vi "Clavier virtuel.vi"(7 "Mode":enum16{"Normal", "Password"}(ring), 8 "error in (no error)":errorcluster, 11 "Str Refnum":refnum<vi>) -> (0 "error out":errorcluster)   [LabVIEW 2012]
doc: "Virutal keyboard ( click on \"-->\" to exit)"
uses:
  <vilib>/Utility/miscctls.llb/LVPointTypeDef.ctl
  <vilib>/Utility/miscctls.llb/LVPositionTypeDef.ctl
panel:
  out "String":string
  out "SHIFT2":bool
  out "SHIFT1":bool
  out "CAPS LOCK":bool
  in  "E3":bool
  in  "E4":bool
  in  "E11":bool
  in  "E6":bool
  in  "E1":bool
  in  "E9":bool
  in  "E5":bool
  in  "E8":bool
  in  "E7":bool
  in  "E12":bool
  in  "E2":bool
  in  "E10":bool
  in  "D3":bool
  in  "D7":bool
  in  "D11":bool
  in  "D1":bool
  in  "D5":bool
  in  "D9":bool
  in  "D4":bool
  in  "D8":bool
  in  "D12":bool
  in  "D2":bool
  in  "D6":bool
  in  "D10":bool
  in  "C2":bool
  in  "C12":bool
  in  "C4":bool
  in  "C10":bool
  in  "C6":bool
  in  "C8":bool
  in  "C1":bool
  in  "C11":bool
  in  "C3":bool
  in  "C9":bool
  in  "C5":bool
  in  "C7":bool
  in  "B1":bool
  in  "B6":bool
  in  "B12":bool
  in  "B11":bool
  in  "B9":bool
  in  "B2":bool
  in  "B5":bool
  in  "B3":bool
  in  "B4":bool
  in  "B7":bool
  in  "B8":bool
  in  "B10":bool
  in  "A12":bool
  in  "A11":bool
  in  "A7":bool
  in  "A9":bool
  in  "A10":bool
  in  "A8":bool
  in  "A6":bool
  in  "A3":bool
  in  "A4":bool
  in  "A5":bool
  in  "A2":bool
  in  "A1":bool
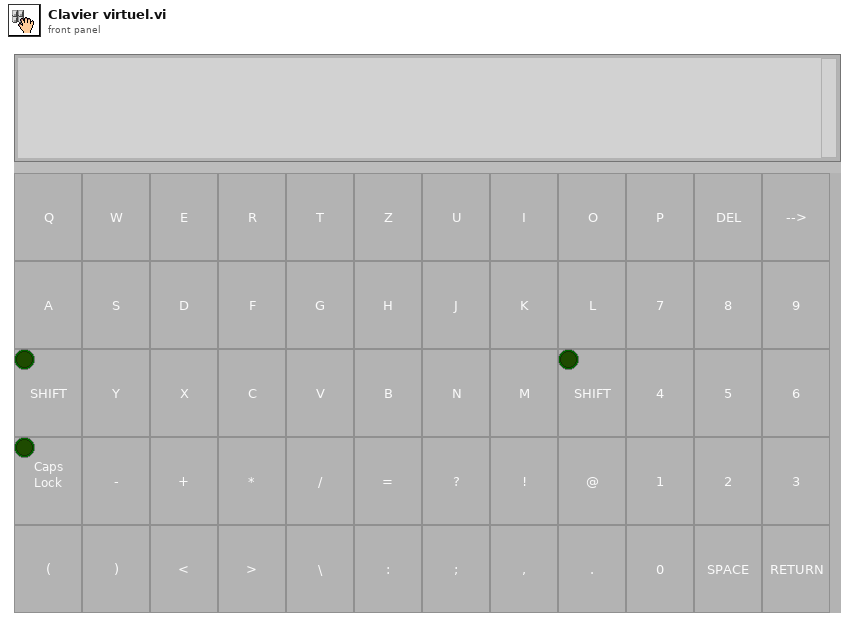
[diagram p1: front panel]
types:
  T1 = typedef "LVPositionTypeDef.ctl" = cluster{"Left":i32, "Top":i32}
  T2 = typedef "LVPointTypeDef.ctl" = cluster{"Horizontal":i16, "Vertical":i16}
  T3 = typedef "LVBoundsTypeDef.ctl" = cluster{"Width":u32, "Height":u32}
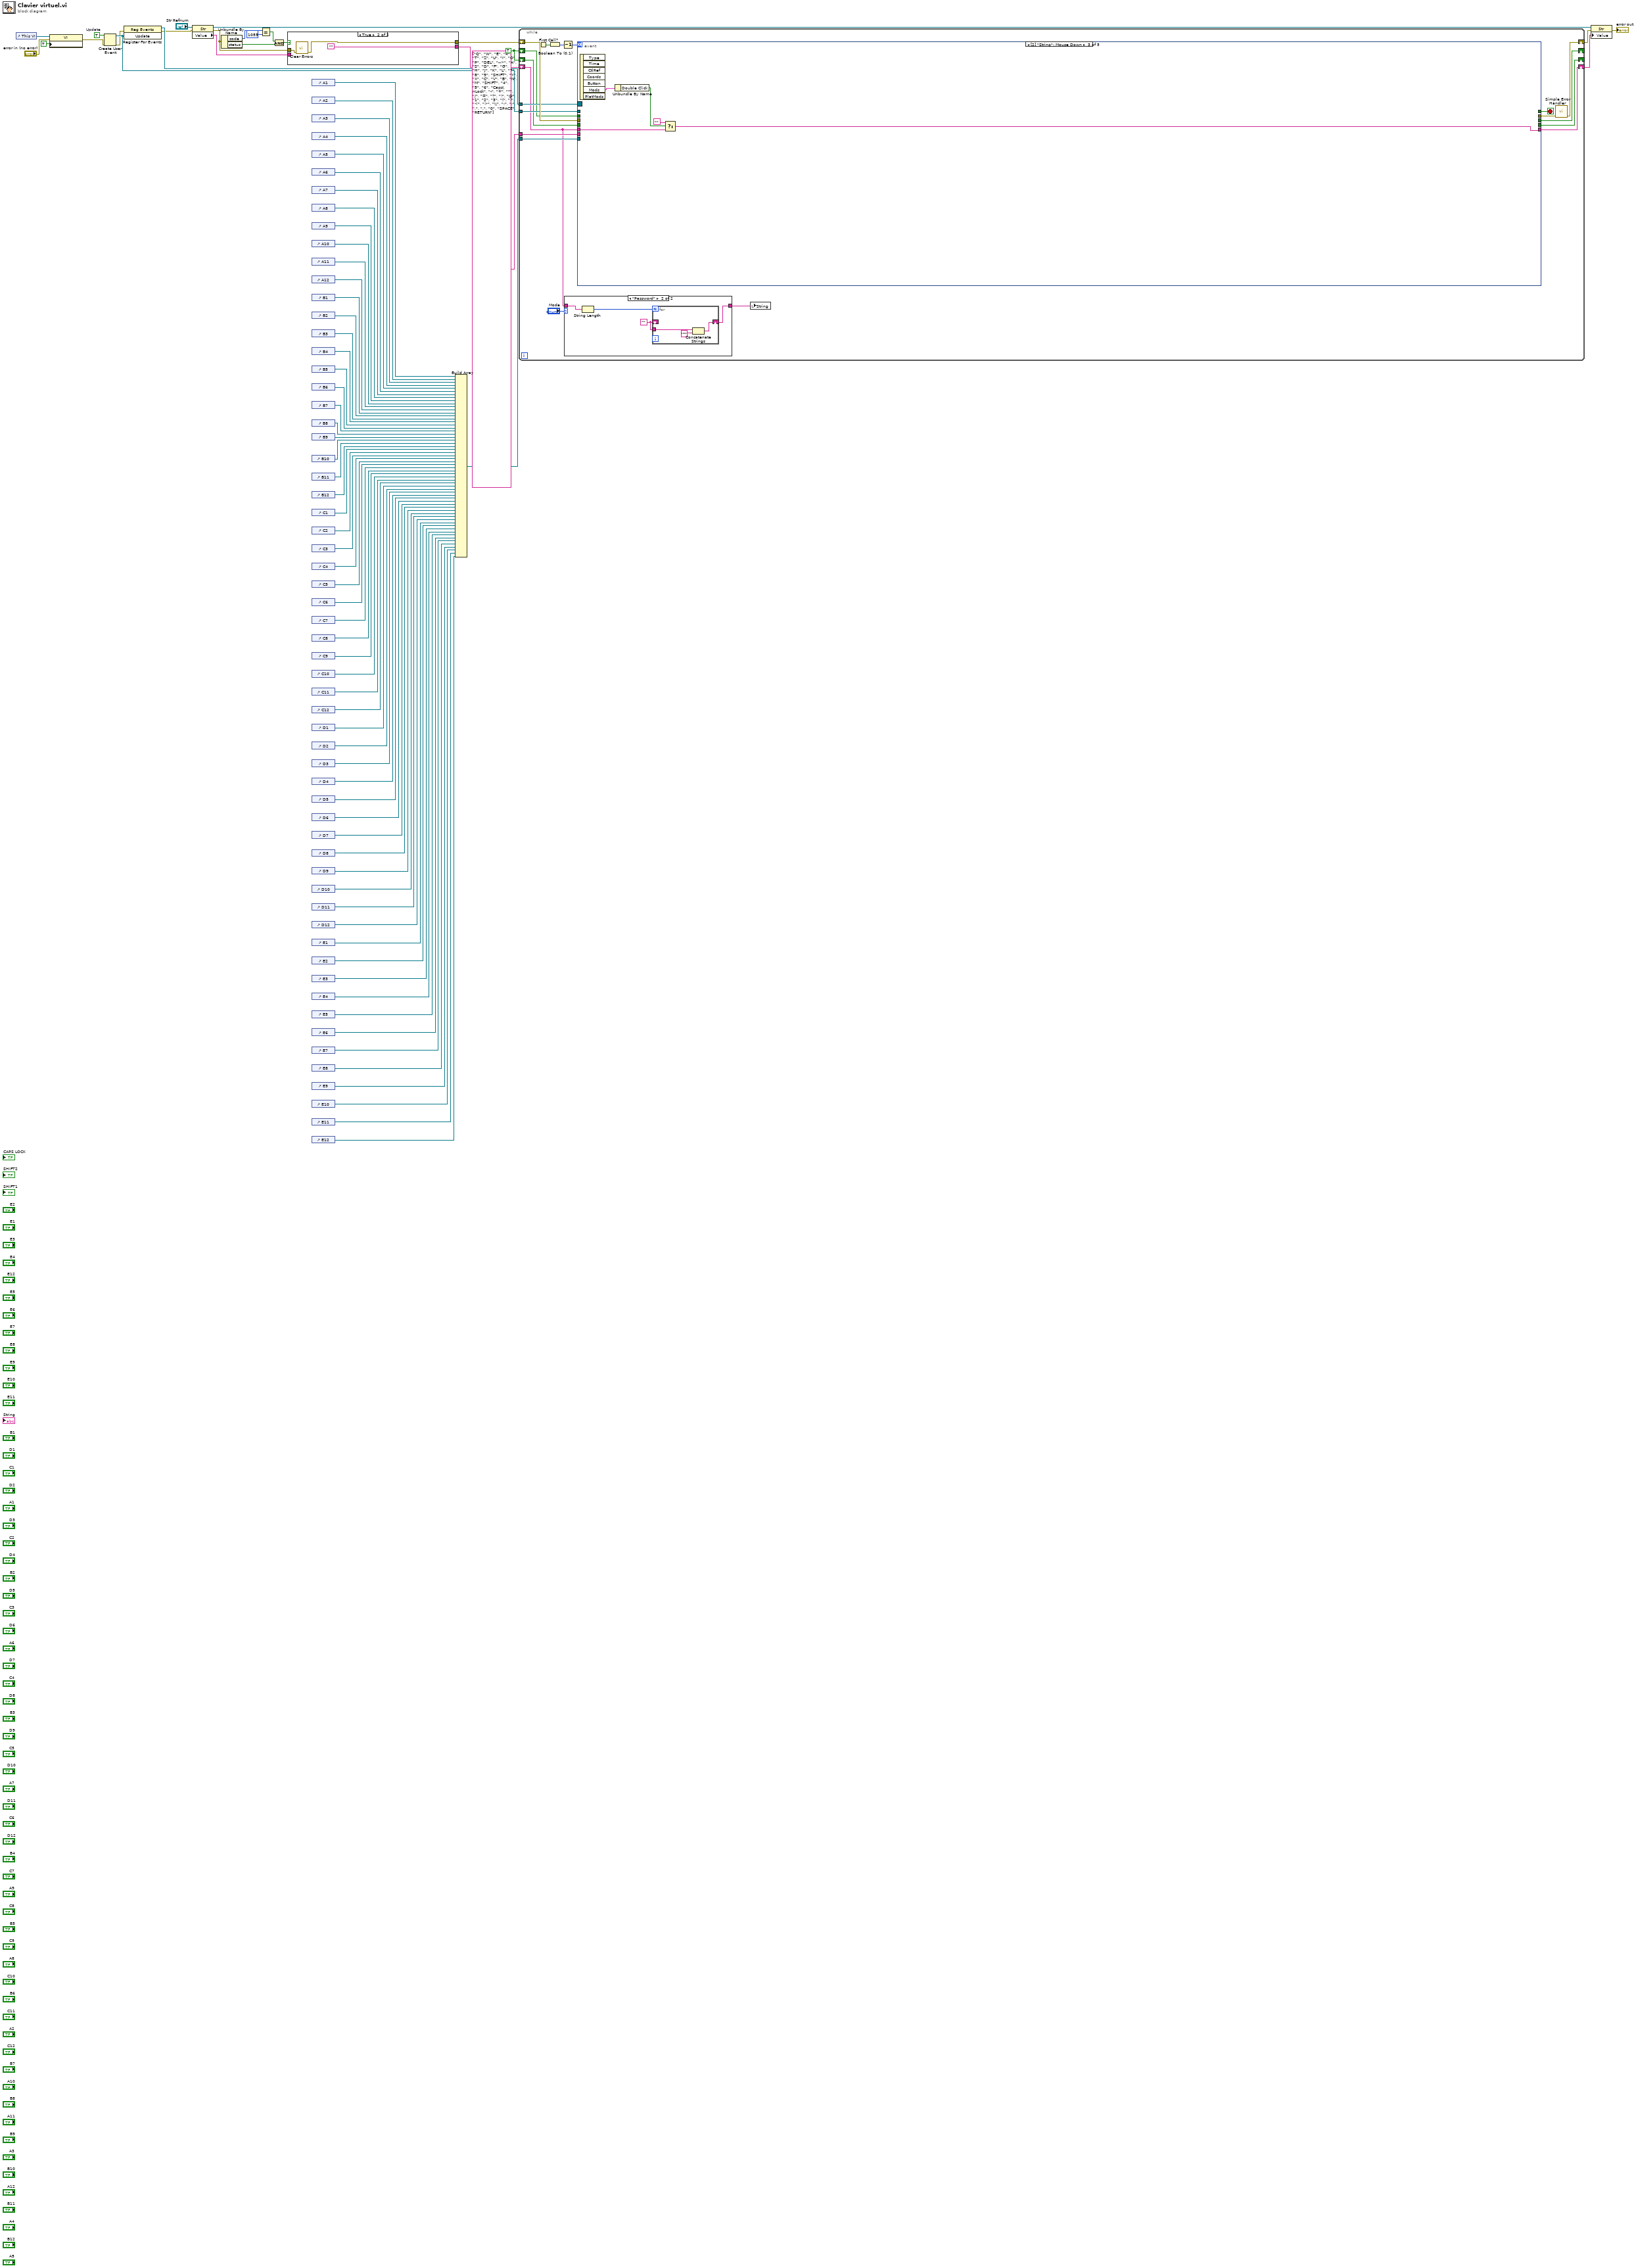
[diagram p0: block diagram]
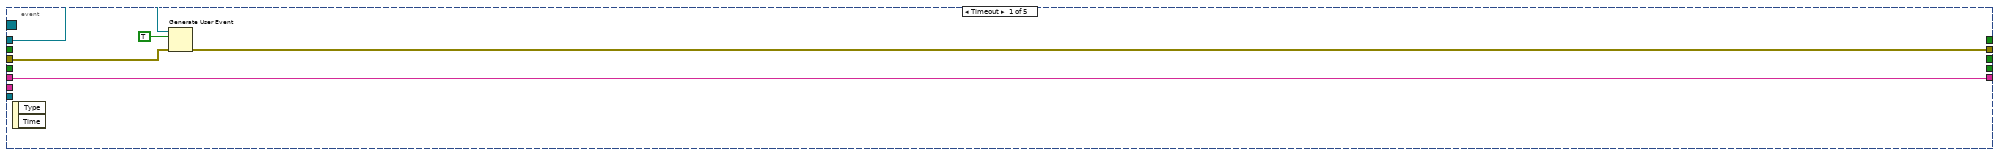
[diagram p4: hidden frame]
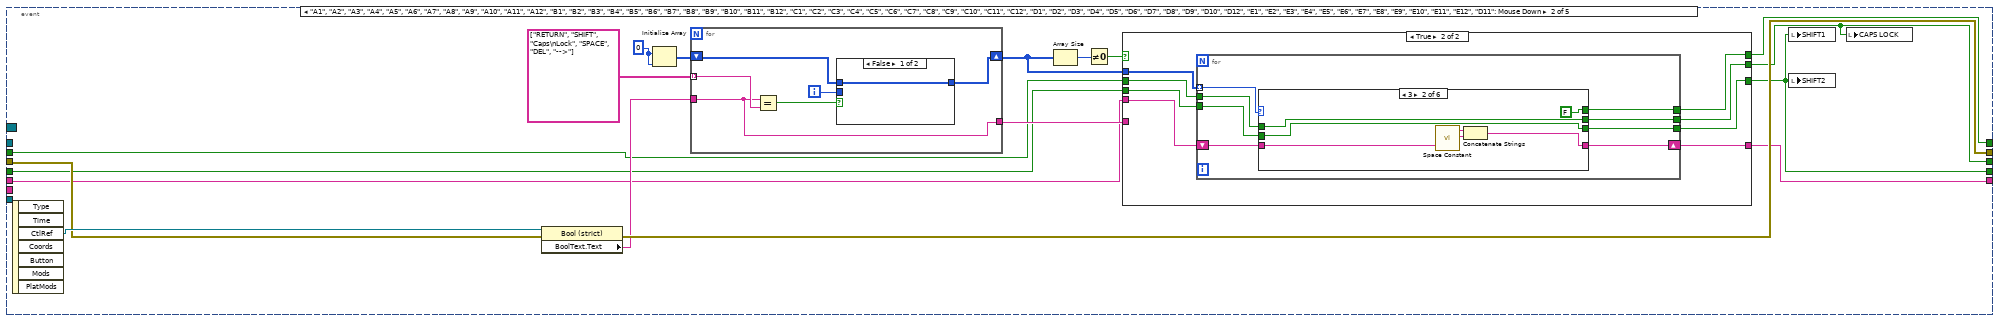
[diagram p5: hidden frame]
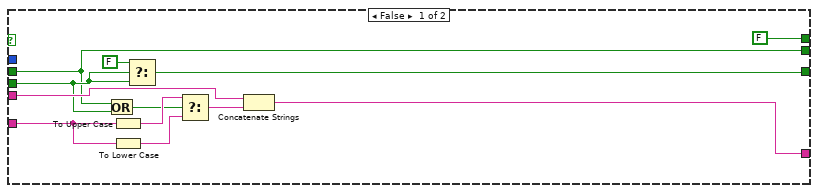
[diagram p6: hidden frame]
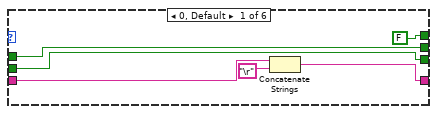
[diagram p7: hidden frame]
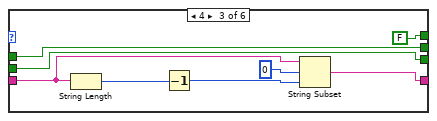
[diagram p8: hidden frame]
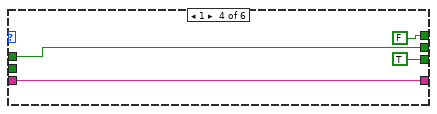
[diagram p9: hidden frame]
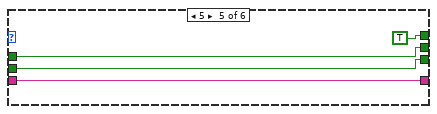
[diagram p10: hidden frame]
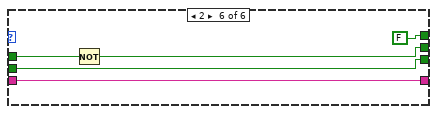
[diagram p11: hidden frame]
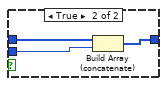
[diagram p12: hidden frame]
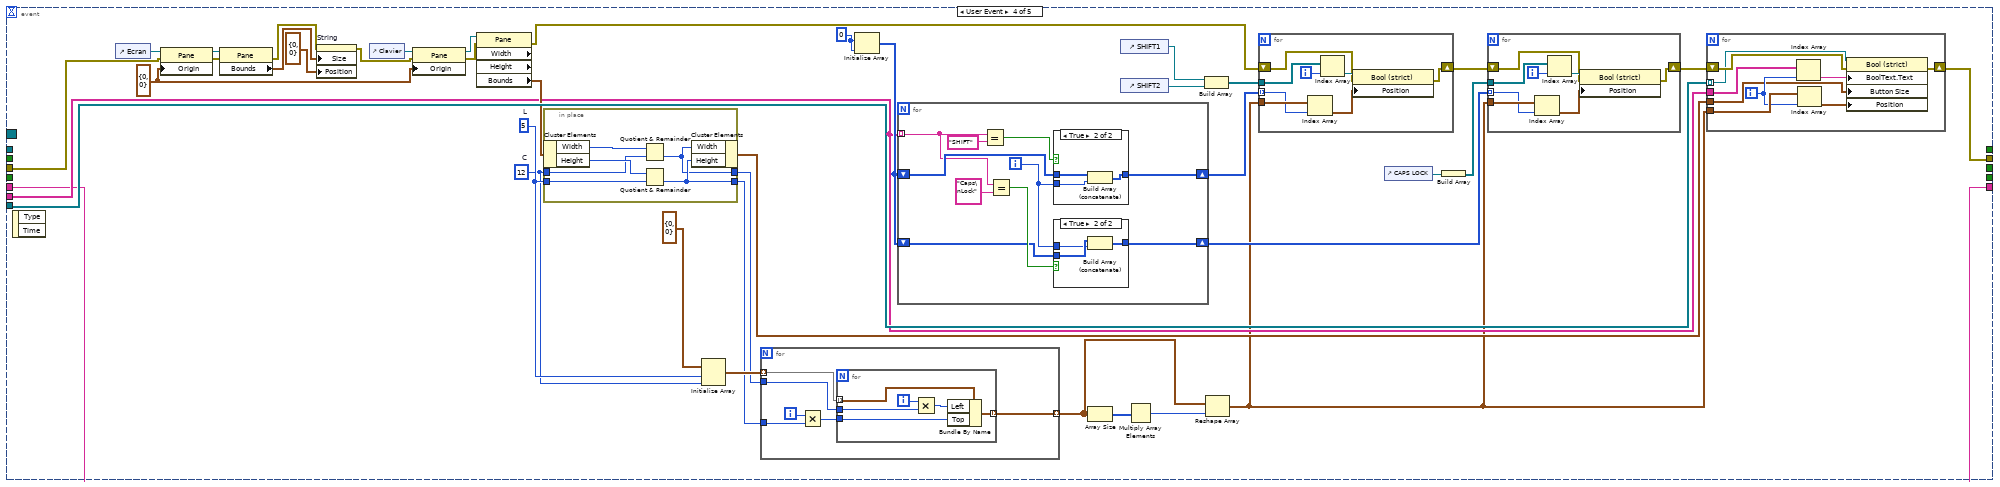
[diagram p13: hidden frame]
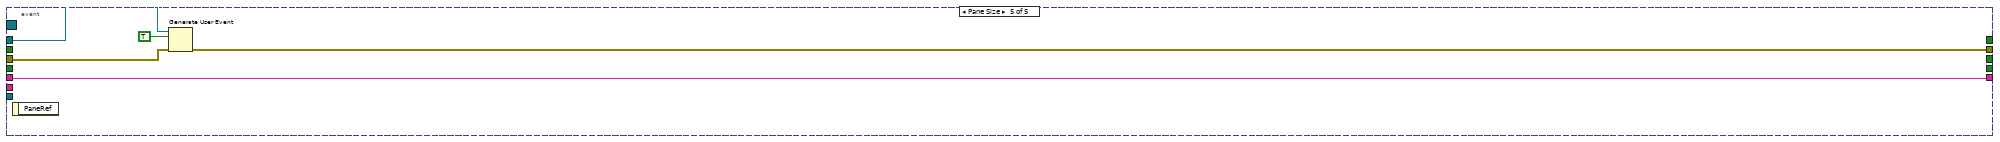
[diagram p16: hidden frame]
diagram:
  w21 = TRUE
  w73 = TRUE  # Update
  n1 = control-ref of="This VI"() -> (w4:refnum<vi>)
  n2 = property class="VI"(reference=w4, error in="error in (no error)", "Front Panel.IsFrontmost"=TRUE ("Front Panel Window:Is Frontmost")) -> (error out=w2:errorcluster)  [unwired: 1 out]
  n3 = Create User Event(user event datatype=w73, error in=w2) -> (user event=w72:refnum<user-event>, error out=w11:errorcluster)
  n4 = register-events(error in=w11, w72) -> (reference out=w71:refnum<event-registration>, error out=w10:errorcluster)  [unwired: 1 in]
  n5 = property class="Str"(reference="Str Refnum", error in=w10) -> (reference out=w16:refnum<vi>, error out=w13:errorcluster, "Value"=w15:string)
  n6 = Unbundle By Name(w13) -> ("code"=w8:i32, "status"=w7:bool)
  n7 = Equal?(x=w8, y=1055) -> (x = y?=w6:bool)
  n8 = And(x=w6, y=w7) -> (x .and. y?=w5:bool)
  n9 = case shown="True" w5 {
    tunnel: w13 -> [w87 w91]
    tunnel: w15 -> [w88 _]
    tunnel: [w88 ""] -> w14
    tunnel: [w87 w90] -> w12
    frame False {
    }
    frame True {
      n10 = call <vilib>:"Clear Errors.vi"("error in (no error)"=w91) -> ("error out"=w90:errorcluster)  [unwired: 6 in]
    }
  }
  n11 = control-ref of="A1"() -> (w82:refnum<vi>)
  n12 = control-ref of="A2"() -> (w83:refnum<vi>)
  n13 = control-ref of="A3"() -> (w84:refnum<vi>)
  n14 = control-ref of="A4"() -> (w85:refnum<vi>)
  n15 = control-ref of="A5"() -> (w86:refnum<vi>)
  n16 = control-ref of="A6"() -> (w81:refnum<vi>)
  n17 = control-ref of="A7"() -> (w80:refnum<vi>)
  n18 = control-ref of="A8"() -> (w79:refnum<vi>)
  n19 = control-ref of="A9"() -> (w78:refnum<vi>)
  n20 = control-ref of="A10"() -> (w77:refnum<vi>)
  n21 = control-ref of="A11"() -> (w76:refnum<vi>)
  n22 = control-ref of="A12"() -> (w75:refnum<vi>)
  n23 = control-ref of="B1"() -> (w69:refnum<vi>)
  n24 = control-ref of="B2"() -> (w68:refnum<vi>)
  n25 = control-ref of="B3"() -> (w67:refnum<vi>)
  n26 = control-ref of="B4"() -> (w66:refnum<vi>)
  n27 = control-ref of="B5"() -> (w65:refnum<vi>)
  n28 = control-ref of="B6"() -> (w64:refnum<vi>)
  n29 = control-ref of="B7"() -> (w63:refnum<vi>)
  n30 = control-ref of="B8"() -> (w62:refnum<vi>)
  n31 = control-ref of="B9"() -> (w61:refnum<vi>)
  n32 = control-ref of="B10"() -> (w60:refnum<vi>)
  n33 = control-ref of="B11"() -> (w59:refnum<vi>)
  n34 = control-ref of="B12"() -> (w58:refnum<vi>)
  n35 = control-ref of="C1"() -> (w57:refnum<vi>)
  n36 = control-ref of="C2"() -> (w56:refnum<vi>)
  n37 = control-ref of="C3"() -> (w55:refnum<vi>)
  n38 = control-ref of="C4"() -> (w54:refnum<vi>)
  n39 = control-ref of="C5"() -> (w53:refnum<vi>)
  n40 = control-ref of="C6"() -> (w52:refnum<vi>)
  n41 = control-ref of="C7"() -> (w51:refnum<vi>)
  n42 = control-ref of="C8"() -> (w50:refnum<vi>)
  n43 = control-ref of="C9"() -> (w49:refnum<vi>)
  n44 = control-ref of="C10"() -> (w48:refnum<vi>)
  n45 = control-ref of="C11"() -> (w47:refnum<vi>)
  n46 = control-ref of="C12"() -> (w46:refnum<vi>)
  n47 = control-ref of="D1"() -> (w45:refnum<vi>)
  n48 = control-ref of="D2"() -> (w44:refnum<vi>)
  n49 = control-ref of="D3"() -> (w43:refnum<vi>)
  n50 = control-ref of="D4"() -> (w42:refnum<vi>)
  n51 = control-ref of="D5"() -> (w41:refnum<vi>)
  n52 = control-ref of="D6"() -> (w40:refnum<vi>)
  n53 = control-ref of="D7"() -> (w39:refnum<vi>)
  n54 = control-ref of="D8"() -> (w38:refnum<vi>)
  n55 = control-ref of="D9"() -> (w37:refnum<vi>)
  n56 = control-ref of="D10"() -> (w36:refnum<vi>)
  n57 = control-ref of="D11"() -> (w35:refnum<vi>)
  n58 = control-ref of="D12"() -> (w34:refnum<vi>)
  n59 = control-ref of="E1"() -> (w33:refnum<vi>)
  n60 = control-ref of="E2"() -> (w32:refnum<vi>)
  n61 = control-ref of="E3"() -> (w31:refnum<vi>)
  n62 = control-ref of="E4"() -> (w30:refnum<vi>)
  n63 = control-ref of="E5"() -> (w29:refnum<vi>)
  n64 = control-ref of="E6"() -> (w28:refnum<vi>)
  n65 = control-ref of="E7"() -> (w27:refnum<vi>)
  n66 = control-ref of="E8"() -> (w26:refnum<vi>)
  n67 = control-ref of="E9"() -> (w25:refnum<vi>)
  n68 = control-ref of="E10"() -> (w24:refnum<vi>)
  n69 = control-ref of="E11"() -> (w23:refnum<vi>)
  n70 = control-ref of="E12"() -> (w22:refnum<vi>)
  n71 = Build Array(w82, w83, w84, w85, w86, w81, w80, w79, w78, w77, w76, w75, w69, w68, w67, w66, w65, w64, w63, w62, w61, w60, w59, w58, w57, w56, w55, w54, w53, w52, w51, w50, w49, w48, w47, w46, w45, w44, w43, w42, w41, w40, w39, w38, w37, w36, w35, w34, w33, w32, w31, w30, w29, w28, w27, w26, w25, w24, w23, w22) -> (w70:refnum<vi>[])
  n72 = while {
    shift-right: [w110] -> w18
    shift-left: w14 -> [w92]
    shift-right: [w95] -> w20
    shift-left: w12 -> [w108]
    tunnel: w70 -> [w104]
    tunnel: string[] ["Q", "W", "E", "R", "T", "Z", "U", "I", "O", "P", "DEL", "-->", "A", "S", "D", "F", "G", "H", "J", "K", "L", "7", "8", "9", "SHIFT", "Y", "X", "C", "V", "B", "N", "M", "SHIFT", "4", "5", "6", "Caps\nLock", "-", "+", "*", "/", "=", "?", "!", "@", "1", "2", "3", "(", ")", "<", ">", "\\", ":", ";", ",", ".", "0", "SPACE", "RETURN"] -> [w103]
    tunnel: w72 -> [w102]
    tunnel: w71 -> [w101]
    shift-right: [w97] -> _
    shift-left: w21 -> [w99]
    shift-right: [w96] -> _
    shift-left: w21 -> [w98]
    stop <- w109 stop-if-true
    n73 = First Call?() -> (First Call?: T/F=w106:bool)
    n74 = Boolean To (0,1)(Boolean=w106) -> (0, 1=w107:i16)
    n75 = Decrement(x=w107) -> (x-1=w105:i16)
    n76 = case shown="\"Password\"" "Mode" {
      tunnel: w92 -> [w111 w115]
      tunnel: [w111 w114] -> w93
      frame "Normal", Default {
      }
      frame "Password" {
        w113 = ""
        n77 = String Length(string=w115) -> (length=w112:i32)
        n78 = for {
          N: w112 -> [_]
          shift-right: [w117] -> w114
          shift-left: w113 -> [_]
          tunnel: w113 -> [w118]
          n79 = Concatenate Strings(w118, "*") -> (w117:string)
        }
      }
    }
    n80 = event shown="[2] \"String\": Mouse Down" {
      selector: w101 -> [_ _ _ _ _]
      dyn-events: _ -> [_ _ _ _ _]
      timeout: w105 -> [_ _ _ _ _]
      tunnel: w92 -> [w119 w128 w215 w218 w319]
      tunnel: [w119 w130 w213 w218 w319] -> w110
      tunnel: [_ w129 _ _ _] -> w109
      tunnel: w108 -> [w121 w140 _ w252 w321]
      tunnel: [w120 w139 _ w250 w320] -> w100
      tunnel: w104 -> [_ _ _ w251 _]
      tunnel: w103 -> [_ _ _ w230 _]
      tunnel: w102 -> [w122 _ _ _ w322]
      tunnel: w99 -> [_ w127 _ _ _]
      tunnel: w98 -> [_ w125 _ _ _]
      tunnel: [_ w126 _ _ _] -> w97
      tunnel: [_ w124 _ _ _] -> w96
      event Timeout {
        n81 = event-data() -> ()  [unwired: 1 in, 2 out]
        n82 = Generate User Event(user event=w122, event data cluster=TRUE ("event data"), error in=w121) -> (error out=w120:errorcluster)  [unwired: 1 out]
      }
      event "A1", "A2", "A3", "A4", "A5", "A6", "A7", "A8", "A9", "A10", "A11", "A12", "B1", "B2", "B3", "B4", "B5", "B6", "B7", "B8", "B9", "B10", "B11", "B12", "C1", "C2", "C3", "C4", "C5", "C6", "C7", "C8", "C9", "C10", "C11", "C12", "D1", "D2", "D3", "D4", "D5", "D6", "D7", "D8", "D9", "D10", "D12", "E1", "E2", "E3", "E4", "E5", "E6", "E7", "E8", "E9", "E10", "E11", "E12", "D11": Mouse Down {
        w138 = 0
        n83 = event-data() -> ("CtlRef"=w141:refnum<vi>)  [unwired: 1 in, 6 out]
        n84 = property class="Bool (strict)"(reference=w141, error in=w140) -> (error out=w139:errorcluster, "BoolText.Text"=w136:string)  [unwired: 1 out]
        n85 = Initialize Array(w138, w138) -> (w135:i32[])
        n86 = for {
          shift-right: [w206] -> w131
          shift-left: w135 -> [w207]
          tunnel: string[] ["RETURN", "SHIFT", "Caps\nLock", "SPACE", "DEL", "-->"] -> [w208] mode=indexing
          tunnel: w136 -> [w203]
          tunnel: [w203] -> w132
          i -> [w204]
          n87 = Equal?(x=w203, y=w208) -> (x = y?=w205:bool)
          n88 = case shown="False" w205 {
            tunnel: w207 -> [w209 w211]
            tunnel: [w209 w212] -> w206
            tunnel: w204 -> [_ w210]
            frame False {
            }
            frame True {
              n89 = Build Array (concatenate)(w211, w210) -> (w212:i32[])
            }
          }
        }
        n90 = Array Size(array=w131) -> (size(s)=w134:i32)
        n91 = Not Equal To 0?(x=w134) -> (x != 0?=w133:bool)
        n92 = case shown="True" w133 {
          tunnel: w132 -> [w152 _]
          tunnel: w128 -> [w149 w158]
          tunnel: [w148 w160] -> w130
          tunnel: w131 -> [_ w161]
          tunnel: [FALSE w159] -> w129
          tunnel: w127 -> [w142 w157]
          tunnel: [w142 w156] -> w126
          tunnel: w125 -> [w143 w155]
          tunnel: [w145 w154] -> w124
          frame False {
            n93 = Or(x=w142, y=w143) -> (x .or. y?=w144:bool)
            n94 = To Upper Case(1:w152) -> (0:w153:string)
            n95 = To Lower Case(string=w152) -> (all lower case string=w151:string)
            n96 = Select(t=FALSE, s=w143, f=w143) -> (s? t:f=w145:bool)
            n97 = Select(t=w153, s=w144, f=w151) -> (s? t:f=w150:string)
            n98 = Concatenate Strings(w149, w150) -> (w148:string)
          }
          frame True {
            n99 = for {
              tunnel: w161 -> [w169] mode=indexing
              shift-right: [w167] -> w160
              shift-left: w158 -> [w168]
              tunnel: [w166] -> w159
              tunnel: w157 -> [w165]
              tunnel: [w164] -> w156
              tunnel: w155 -> [w163]
              tunnel: [w162] -> w154
              n100 = case shown="3" w169 {
                tunnel: w168 -> [w175 w181 w185 w193 w197 w202]
                tunnel: [w174 w180 w186 w193 w197 w202] -> w167
                tunnel: [FALSE FALSE FALSE FALSE TRUE FALSE] -> w166
                tunnel: w165 -> [w171 w177 w183 w191 w195 w200]
                tunnel: [w171 w177 w183 w191 w195 w198] -> w164
                tunnel: w163 -> [w170 w176 w182 _ w194 w199]
                tunnel: [w170 w176 w182 TRUE w194 w199] -> w162
                frame 0, Default {
                  n101 = Concatenate Strings(w175, "\r") -> (w174:string)
                }
                frame 3 {
                  n102 = call <vilib>:"Space Constant.vi"() -> ("String"=w179:string)
                  n103 = Concatenate Strings(w181, w179) -> (w180:string)
                }
                frame 4 {
                  n104 = String Length(string=w185) -> (length=w188:i32)
                  n105 = Decrement(x=w188) -> (x-1=w189:i32)
                  n106 = String Subset(string=w185, offset (0)=0, length (rest)=w189) -> (substring=w186:string)
                }
                frame 1 {
                }
                frame 5 {
                }
                frame 2 {
                  n107 = Not(x=w200) -> (.not. x?=w198:bool)
                }
              }
            }
          }
        }
        n108 = local write "SHIFT1"(w124) -> ()
        n109 = local write "SHIFT2"(w124) -> ()
        n110 = local write "CAPS LOCK"(w126) -> ()
      }
      event "String": Mouse Down {
        n111 = event-data() -> ("Mods"=w217:cluster{"Double Click":bool, "Menu Key":bool})  [unwired: 1 in, 6 out]
        n112 = Unbundle By Name(w217) -> ("Double Click"=w216:bool)
        n113 = Select(t="", s=w216, f=w215) -> (s? t:f=w213:string)
      }
      event User Event {
        w231 = 0
        w233 = 12  # C
        w236 = 5  # L
        w255 = T2 {"Horizontal"=0, "Vertical"=0} ("Origin")
        n114 = event-data() -> ()  [unwired: 1 in, 2 out]
        n115 = control-ref of="Ecran"() -> (w257:refnum<vi>)
        n116 = property class="Pane"(reference=w257, error in=w252, "Origin"=w255) -> (reference out=w249:refnum<vi>, error out=w247:errorcluster)
        n117 = property class="Pane"(reference=w249, error in=w247) -> (error out=w246:errorcluster, "Bounds"=w253:T3)  [unwired: 1 out]
        n118 = property on="String" class="Str"(error in=w246, "Size"=w253, "Position"=T1 {"Left"=0, "Top"=0}) -> (error out=w245:errorcluster)  [unwired: 1 in, 1 out]
        n119 = control-ref of="Clavier"() -> (w256:refnum<vi>)
        n120 = property class="Pane"(reference=w256, error in=w245, "Origin"=w255) -> (reference out=w248:refnum<vi>, error out=w244:errorcluster)
        n121 = property class="Pane" props=["Width", "Height", "Bounds"](reference=w248, error in=w244) -> (error out=w224:errorcluster, "Bounds"=w243:T3)  [unwired: 3 out]
        n122 = in-place {
          in-place-border: [w307] -> w235
          in-place-border: [w306] -> w234
          in-place-border: w236 -> [w305]
          in-place-border: w233 -> [w304]
          n123 = in-place-cluster #1(w243) -> ("Width"=w309:u32, "Height"=w308:u32)
          n124 = Quotient & Remainder(x=w309, y=w304) -> (floor(x/y)=w306:u32)  [unwired: 1 out]
          n125 = Quotient & Remainder(x=w308, y=w305) -> (floor(x/y)=w307:u32)  [unwired: 1 out]
          n126 = in-place-cluster #1("Width"=w306, "Height"=w307) -> (w242:T3)
        }
        n127 = Initialize Array(T1 {"Left"=0, "Top"=0} ("Position"), w236, w233) -> (w238:T1[][])
        n128 = for {
          tunnel: w238 -> [w297] mode=indexing
          tunnel: [w296] -> w239 mode=indexing
          tunnel: w235 -> [w295]
          tunnel: w234 -> [w292]
          i -> [w294]
          n129 = Multiply(x=w294, y=w295) -> (x*y=w293:u32)
          n130 = for {
            tunnel: w297 -> [w303] mode=indexing
            tunnel: [w302] -> w296 mode=indexing
            tunnel: w293 -> [w301]
            tunnel: w292 -> [w298]
            i -> [w300]
            n131 = Multiply(x=w300, y=w298) -> (x*y=w299:u32)
            n132 = Bundle By Name(cluster=w303, "Left"=w299, "Top"=w301) -> (w302:T1)
          }
        }
        n133 = Initialize Array(w231, w231) -> (w232:i32[])
        n134 = for {
          tunnel: w230 -> [w278] mode=indexing
          shift-right: [w280] -> w225
          shift-left: w232 -> [w281]
          shift-right: [w275] -> w220
          shift-left: w232 -> [w276]
          i -> [w274]
          n135 = Equal?(x=w278, y="SHIFT") -> (x = y?=w282:bool)
          n136 = Equal?(x=w278, y="Caps\nLock") -> (x = y?=w277:bool)
          n137 = case shown="True" w282 {
            tunnel: w281 -> [w288 w291]
            tunnel: [w288 w290] -> w280
            tunnel: w274 -> [_ w289]
            frame False {
            }
            frame True {
              n138 = Build Array (concatenate)(w291, w289) -> (w290:i32[])
            }
          }
          n139 = case shown="True" w277 {
            tunnel: w276 -> [w284 w287]
            tunnel: [w284 w286] -> w275
            tunnel: w274 -> [_ w285]
            frame False {
            }
            frame True {
              n140 = Build Array (concatenate)(w287, w285) -> (w286:i32[])
            }
          }
        }
        n141 = Array Size(array=w239) -> (size(s)=w240:i32[])
        n142 = control-ref of="SHIFT1"() -> (w229:refnum<vi>)
        n143 = control-ref of="SHIFT2"() -> (w228:refnum<vi>)
        n144 = Multiply Array Elements(1:w240) -> (0:w241:i32)
        n145 = Build Array(w229, w228) -> (w226:refnum<vi>[])
        n146 = Reshape Array(w239, w241) -> (w219:T1[])
        n147 = for {
          tunnel: w226 -> [w270]
          tunnel: w219 -> [w272]
          tunnel: w225 -> [w271] mode=indexing
          shift-right: [w266] -> w223
          shift-left: w224 -> [w267]
          i -> [w268]
          n148 = Index Array(array=w272, index=w271) -> (element=w273:T1)
          n149 = Index Array(array=w270, index=w268) -> (element=w269:refnum<vi>)
          n150 = property class="Bool (strict)"(reference=w269, error in=w267, "Position"=w273) -> (error out=w266:errorcluster)  [unwired: 1 out]
        }
        n151 = control-ref of="CAPS LOCK"() -> (w227:refnum<vi>)
        n152 = Build Array(w227) -> (w222:refnum<vi>[])
        n153 = for {
          tunnel: w222 -> [w262]
          tunnel: w219 -> [w264]
          tunnel: w220 -> [w263] mode=indexing
          shift-right: [w258] -> w221
          shift-left: w223 -> [w259]
          i -> [w260]
          n154 = Index Array(array=w264, index=w263) -> (element=w265:T1)
          n155 = Index Array(array=w262, index=w260) -> (element=w261:refnum<vi>)
          n156 = property class="Bool (strict)"(reference=w261, error in=w259, "Position"=w265) -> (error out=w258:errorcluster)  [unwired: 1 out]
        }
        n157 = for {
          tunnel: w251 -> [w314] mode=indexing
          shift-right: [w317] -> w250
          shift-left: w221 -> [w318]
          tunnel: w230 -> [w316]
          tunnel: w219 -> [w313]
          tunnel: w242 -> [w311]
          i -> [w312]
          n158 = Index Array(array=w316, index=w312) -> (element=w315:string)
          n159 = Index Array(array=w313, index=w312) -> (element=w310:T1)
          n160 = property class="Bool (strict)"(reference=w314, error in=w318, "BoolText.Text"=w315, "Button Size"=w311, "Position"=w310) -> (error out=w317:errorcluster)  [unwired: 1 out]
        }
      }
      event Pane Size {
        n161 = event-data() -> ()  [unwired: 1 in, 1 out]
        n162 = Generate User Event(user event=w322, event data cluster=TRUE ("event data"), error in=w321) -> (error out=w320:errorcluster)  [unwired: 1 out]
      }
    }
    n163 = local write "String"(w93) -> ()
    n164 = call <vilib>:"Simple Error Handler.vi"("error in (no error)"=w100) -> ("error out"=w95:errorcluster)  [unwired: 4 in, 4 out]
  }
  n165 = property class="Str"(reference=w16, error in=w20, "Value"=w18) -> (error out=→"error out":errorcluster)  [unwired: 1 out]
